vi "Set Curr Mode.vi"(8 "error in (no error)":errorcluster, 9 "Curr Loop Cmd Q":refnum<queue>, 11 "Async Data in":T1={"Hardware"={"Switch Device"="", "DMM Device"="", "DMM -> Switch Trigger"=0, "Switch -> DMM Trigger"=0, "Sample Interval (sec)"=0.0, "Current Samples"=0, "Current Limit"=1.2, "Current Resolution"=5.5, "Auto-Read"=FALSE, "Keep Values"=FALSE}, "Communication"={"Status Q"=refnum, "Command Q"=refnum, "Voltage FIFO"=refnum, "Voltage Buffer"=[], "Current FIFO"=refnum, "Current Buffer"=[], "Async Events"=refnum}} {"Hardware"."Current Resolution" items=["3 1/2"=3.5, "4 1/2"=4.5, "5 1/2"=5.5, "6 1/2"=6.5, "7 1/2"=7.5]; "Hardware"."Sample Interval (sec)" format="%.2f"}) -> (0 "error out":errorcluster)   [LabVIEW 2011, in "Switch-DMM Custom Device.lvlib"]
uses:
  Switch-DMM Custom Device.lvlib
  Controls/Async Data.ctl
  Controls/Hardware.ctl
  <instrlib>/niDMM/nidmm.llb/niDMM Resolution in Digits.ctl
  Controls/Communication.ctl
  Controls/Async Status.ctl
  Controls/Async State.ctl
  Controls/Async Command.ctl
  Controls/Async Events.ctl
  Controls/Cur Loop Cmd.ctl
  <instrlib>/niSwitch/niSwitch.LLB/niSwitch Connect Channels (Single).vi
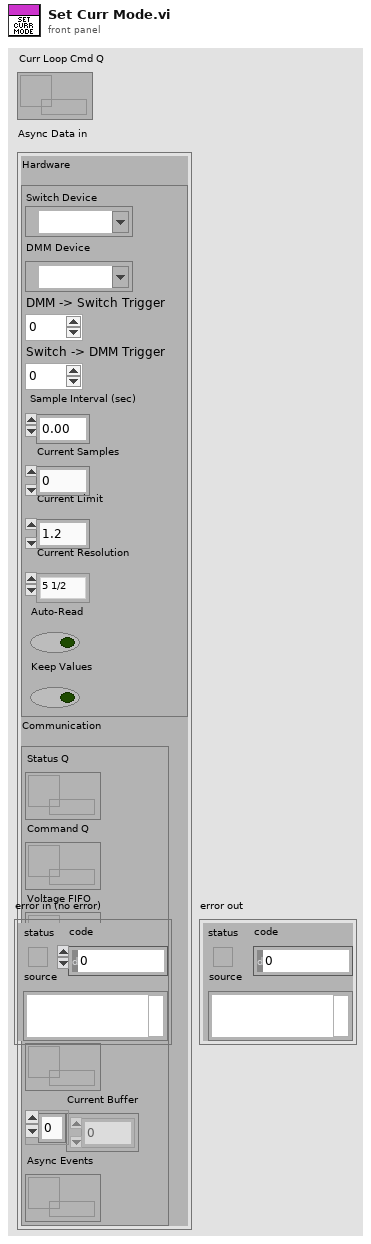
[diagram p1: front panel]
types:
  T1 = typedef "Switch-DMM Custom Device.lvlib/Async Data.ctl" = cluster{"Hardware":T2, "Communication":T4}
  T2 = typedef "Switch-DMM Custom Device.lvlib/Hardware.ctl" = cluster{"Switch Device":refnum<k15>, "DMM Device":refnum<k15>, "DMM -> Switch Trigger":u16, "Switch -> DMM Trigger":u16, "Sample Interval (sec)":dbl, "Current Samples":i32, "Current Limit":dbl, "Current Resolution":T3, "Auto-Read":bool, "Keep Values":bool}
  T3 = typedef "niDMM Resolution in Digits.ctl" = dbl
  T4 = typedef "Switch-DMM Custom Device.lvlib/Communication.ctl" = cluster{"Status Q":refnum<queue>, "Command Q":refnum<queue>, "Voltage FIFO":refnum<k33>, "Voltage Buffer":dbl[], "Current FIFO":refnum<k33>, "Current Buffer":dbl[], "Async Events":refnum<queue>}
  T5 = typedef "Switch-DMM Custom Device.lvlib/Cur Loop Cmd.ctl" = enum16{"None", "Start", "Stop", "Exit"}
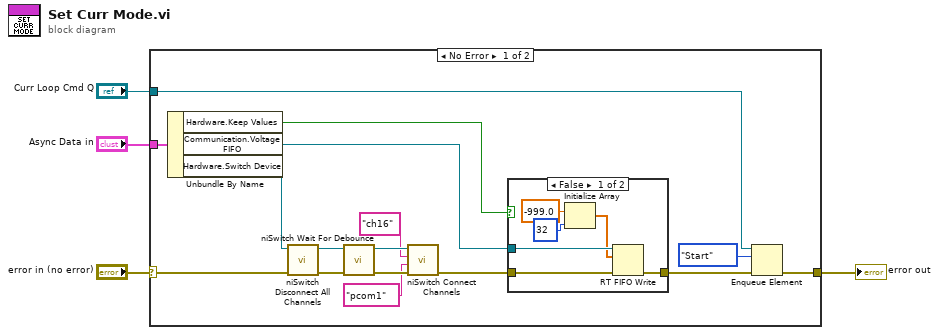
[diagram p0: block diagram]
diagram:
  n1 = case shown="No Error" "error in (no error)" {
    selector: "error in (no error)" -> [w9 w28]
    tunnel: "Async Data in" -> [w19 _]
    tunnel: [w18 w28] -> w3
    tunnel: "Curr Loop Cmd Q" -> [w10 _]
    frame No Error {
      n2 = Unbundle By Name(w19) -> ("Hardware.Keep Values"=w7:bool, "Communication.Voltage FIFO"=w8:refnum<k33>, "Hardware.Switch Device"=w20:refnum<k15>)
      n3 = call <instrlib>:"niSwitch Disconnect All Channels.vi"("error in (no error)"=w9, "instrument handle"=w20) -> ("error out"=w16:errorcluster, "instrument handle out"=w17:refnum<k15>)  [unwired: 8 in]
      n4 = call <instrlib>:"niSwitch Wait For Debounce.vi"("error in (no error)"=w16, "instrument handle"=w17) -> ("error out"=w14:errorcluster, "instrument handle out"=w15:refnum<k15>)  [unwired: 8 in]
      n5 = call-poly <instrlib>:"niSwitch Connect Channels.vi"("error in (no error)"=w14, "channel 2"="pcom1", "channel 1"="ch16", "instrument handle"=w15) -> ("error out"=w6:errorcluster)  [unwired: 6 in, 1 out]
      n6 = case shown="False" w7 {
        tunnel: w6 -> [w26 w27]
        tunnel: w8 -> [w25 _]
        tunnel: [w24 w27] -> w5
        frame False {
          n7 = Initialize Array(-999.0, 32 ("dimension size")) -> (w21:dbl[])
          n8 = RT FIFO Write(0:w25, 1:w21, 3:w26) -> (11:w24:errorcluster)  [unwired: 2 in, 3 out]
        }
        frame True {
        }
      }
      n9 = Enqueue Element(queue=w10, element=Cur_Loop_Cmd."Start", error in (no error)=w5) -> (error out=w18:errorcluster)  [unwired: 1 in, 2 out]
    }
    frame Error {
    }
  }
  "error out" <- w3
